vi "mod_Kaiser FIR Filter Design.vi"(2 "Stop Attenuation":dbl format="%.2f", 3 "sampling freq: fs":dbl=1.0 format="%.2f", 4 "high cutoff freq: fh":dbl=0.45 format="%.2f", 5 "low cutoff freq: fl":dbl=0.125 format="%.2f") -> (0 "Estimated Taps":i32, 1 "h":dbl[](array[numeric]) format="%.2f")   [LabVIEW 2020, in "niAMT.lvlib"]
uses:
  <vilib>/addons/Modulation/niAMT.lvlib
  <vilib>/Analysis/4window.llb/windowTd.ctl
  <vilib>/Analysis/NI_AALBase.lvlib
  <vilib>/Analysis/NI_AALPro.lvlib
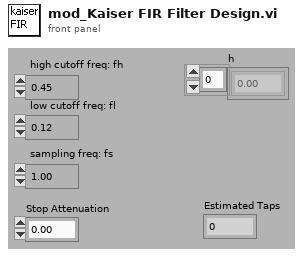
[diagram p1: front panel]
types:
  T1 = typedef "NI_AALPro.lvlib/windowTd.ctl" = u32
  T2 = enum32{"Lowpass", "Highpass", "Bandpass", "Bandstop"}
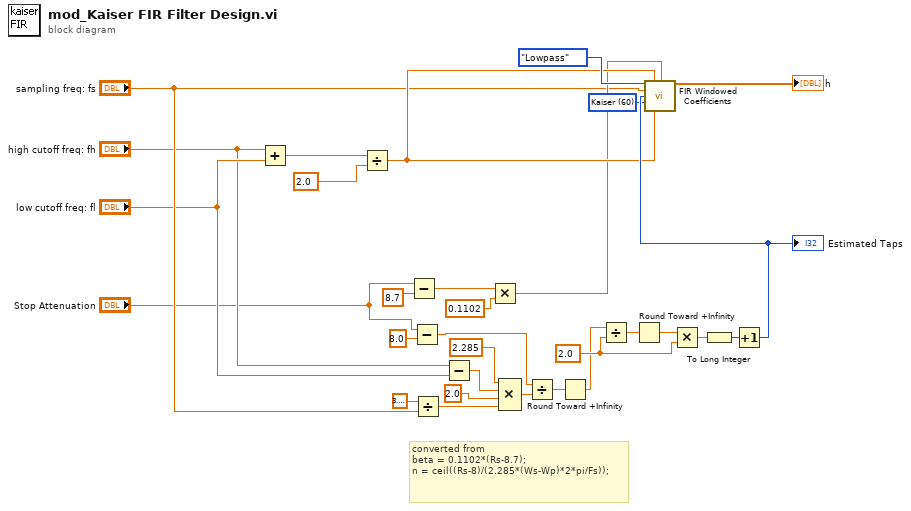
[diagram p0: block diagram]
diagram:
  w20 = T1 60 items=["Rectangle"=0, "Hanning"=1, "Hamming"=2, "Blackman-Harris"=3, "Exact Blackman"=4, "Blackman"=5, "Flat Top"=6, "4 Term B-Harris "=7, "7 Term B-Harris"=8, "Low Sidelobe"=9, "Blackman Nuttall"=11, "Triangle"=30, "Bartlett-Hanning"=31, "Bohman"=32, "Parzen"=33, "Welch"=34, "Kaiser"=60, "Dolph-Chebyshev"=61, "Gaussian"=62] ("window")
  w28 = 2.0 ("y")
  # "converted from \nbeta = 0.1102*(Rs-8.7);\nn = ceil((Rs-8)/(2.285*(Ws-Wp)*2*pi/Fs));"
  n1 = Add(x="high cutoff freq: fh", y="low cutoff freq: fl") -> (x+y=w30:dbl)
  n2 = Divide(x=w30, y=2.0) -> (x/y=w19:dbl)
  n3 = Subtract(x="Stop Attenuation", y=8.7) -> (x-y=w17:dbl)
  n4 = Subtract(x="Stop Attenuation", y=8.0) -> (x-y=w14:dbl)
  n5 = Divide(x=3.141592653589793, y="sampling freq: fs") -> (x/y=w9:dbl)
  n6 = Subtract(x="high cutoff freq: fh", y="low cutoff freq: fl") -> (x-y=w11:dbl)
  n7 = Multiply(x=w17, y=0.1102) -> (x*y=w5:dbl)
  n8 = Compound Arithmetic op=MULTIPLY(2.285 ("value"), w11, 2.0 ("value"), w9) -> (w8:dbl)
  n9 = Divide(x=w14, y=w8) -> (x/y=w7:dbl)
  n10 = Round Toward +Infinity(x=w7) -> (ceil(x): smallest int >= x=w6:dbl)
  n11 = Divide(x=w6, y=w28) -> (x/y=w25:dbl)
  n12 = Round Toward +Infinity(x=w25) -> (ceil(x): smallest int >= x=w24:dbl)
  n13 = Multiply(x=w24, y=w28) -> (x*y=w27:dbl)
  n14 = To Long Integer(number=w27) -> (32bit integer=w26:i32)
  n15 = Increment(x=w26) -> (x+1=w21:i32)
  "Estimated Taps" <- w21
  n16 = call <vilib>:"FIR Windowed Coefficients.vi"("filter type"=T2."Lowpass", "high cutoff freq: fh"=w19, "window parameter"=w5, "sampling freq: fs"="sampling freq: fs", "taps"=w21, "window"=w20, "low cutoff freq: fl"=w19) -> ("FIR Windowed Coefficients"=→"h":dbl[])  [unwired: 7 in, 1 out]
